vi "Read window.open.vi"(8 "error in (no error)":errorcluster, 11 "rqcBob in":refnum<class "rqcBob.lvclass">) -> (0 "error out":errorcluster, 2 "window.open":u16, 3 "rqcBob out":refnum<class "rqcBob.lvclass">)   [LabVIEW 2019, in "rqcBob.lvclass"]
uses:
  rqcBob.lvclass
  rqcBob.lvclass/rqcBob.ctl
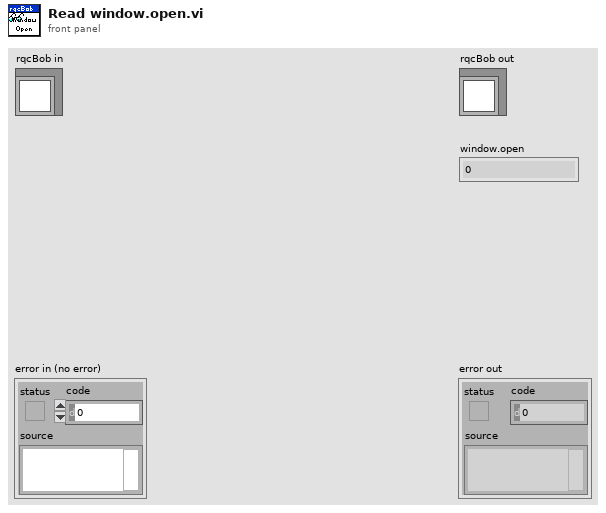
[diagram p1: front panel]
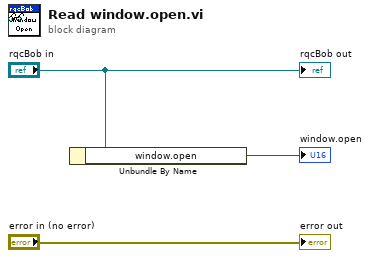
[diagram p0: block diagram]
diagram:
  n1 = Unbundle By Name("rqcBob in") -> ("window.open"=→"window.open":u16)
  "error out" <- "error in (no error)"
  "rqcBob out" <- "rqcBob in"
